vi "ExtractArchivedSpectrum.vi"() -> ()   [LabVIEW 2009]
uses:
  tango_lv8/tango_vi.llb/avToDoubleSpectrumAv.vi
panel:
  out "Intensity Chart":dbl[][](graph)
  out "timestamps":dbl[](array[numeric])
  out "archived sprectra":dbl[][](array[numeric])
  in  "sampling":string="MINUTE"
  in  "to_date":string="2010-02-02 00:00:00"
  in  "from_date":string="2010-02-01 00:00:00"
  in  "archived_attr_name":string="ANS-C03/DG/DCCT/current"
  in  "db_extractor_dev_name":string="archiving/hdbextractor/1"
  out "error stack":string[](array[string])
  out "error code":i32
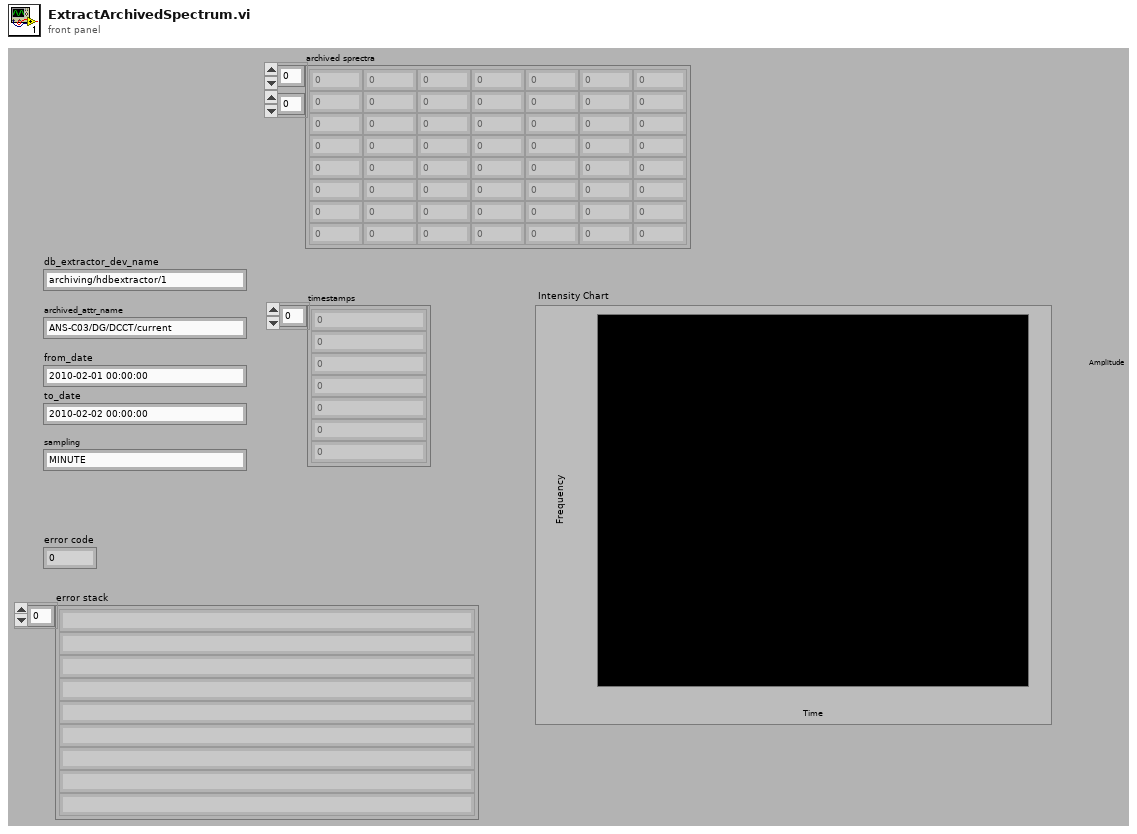
[diagram p1: front panel]
types:
  T1 = cluster{"device name":string, "attribute name":string, "quality value":i16, "quality string":string, "timestamp":dbl, "dim. x":i32, "dim. y":i32, "value":u8[], "error code":i32, "error stack":string[], "data type":enum16{"SCA_STATE", "SCA_STRING", "SPE_STRING", "IMG_STRING", "SCA_BOOLEAN", "SPE_BOOLEAN", "IMG_BOOLEAN", "SCA_UCHAR", "SPE_UCHAR", "IMG_UCHAR", "SCA_SHORT", "SPE_SHORT", "IMG_SHORT", "SCA_USHORT", "SPE_USHORT", "IMG_USHORT", "SCA_LONG", "SPE_LONG", "IMG_LONG", "SCA_ULONG", "SPE_ULONG", "IMG_ULONG", "SCA_FLOAT", "SPE_FLOAT", "IMG_FLOAT", "SCA_DOUBLE", "SPE_DOUBLE", "IMG_DOUBLE", "UNKNOWN_TYPE"}}[]
  T2 = cluster{"device name":string, "attribute name":string, "quality value":i16, "quality string":string, "timestamp":dbl, "dim. x":i32, "dim. y":i32, "value":dbl[], "error code":i32, "error stack":string[]}
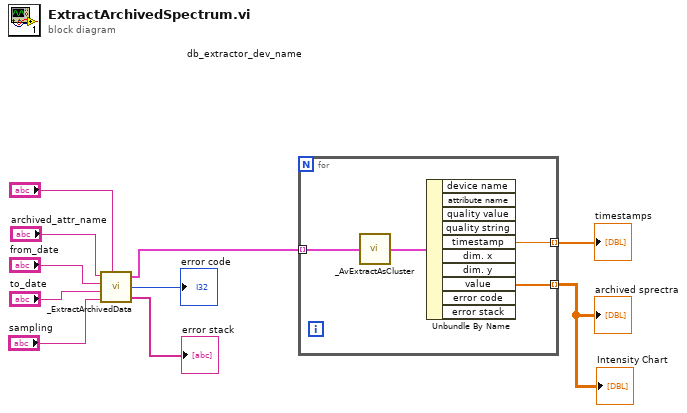
[diagram p0: block diagram]
diagram:
  n1 = call "_ExtractArchivedData.vi"("archived_attr_name"="archived_attr_name", "from_date"="from_date", "to_date"="to_date", "sampling"="sampling", "db_extractor_dev_name"="db_extractor_dev_name") -> ("values"=w3:T1, "error code"=→"error code":i32, "error stack"=→"error stack":string[])
  n2 = for {
    tunnel: w3 -> [w14] mode=indexing
    tunnel: [w12] -> w2 mode=indexing
    tunnel: [w11] -> w1 mode=indexing
    n3 = call-poly "_AvExtractAsCluster.vi"("attribute value"=w14) -> ("av"=w13:T2)
    n4 = Unbundle By Name(w13) -> ("timestamp"=w12:dbl, "value"=w11:dbl[])  [unwired: 8 out]
  }
  "archived sprectra" <- w1
  "timestamps" <- w2
  "Intensity Chart" <- w1
